vi "MC-21C Driver_simple.vi"(8 "Step":string="200", 9 "Operation":enum16{"forward", "backward", "stop"}(ring), 10 "Address":u8=1, 11 "Peristaltic Pump COM":refnum<visa-resource-name>="COM3") -> (2 "Write buffer":string)   [LabVIEW 2023]
panel:
  out "Read buffer":string
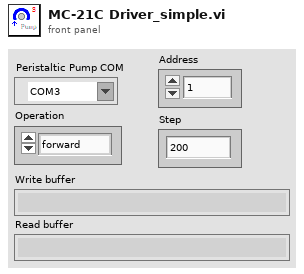
[diagram p1: front panel]
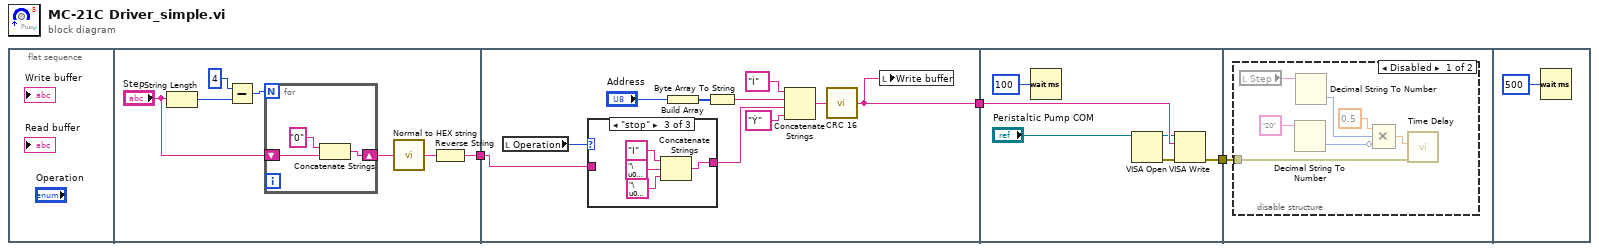
[diagram p0: block diagram]
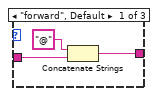
[diagram p2: hidden frame]
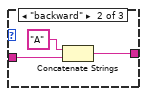
[diagram p3: hidden frame]
diagram:
  n1 = flat-sequence {
    tunnel: [w4] -> w3
    tunnel: w3 -> [w23]
    tunnel: [w14] -> w2
    tunnel: w2 -> [w37]
    tunnel: [w34] -> w1
    tunnel: w1 -> [w40]
    frame #0 {
    }
    frame #1 {
      n2 = String Length(string="Step") -> (length=w7:i32)
      n3 = Subtract(x=4, y=w7) -> (x-y=w8:i32)
      n4 = for {
        N: w8 -> [_]
        shift-right: [w11] -> w10
        shift-left: "Step" -> [w13]
        n5 = Concatenate Strings("0" ("string"), w13) -> (w11:string)
      }
      n6 = call "Normal to HEX string.vi"("input normal string"=w10) -> ("output HEX string"=w6:string)
      n7 = Reverse String(1:w6) -> (0:w4:string)
    }
    frame #2 {
      n8 = local read "Operation"() -> (w18:enum16{"forward", "backward", "stop"})
      n9 = case shown="\"stop\"" w18 {
        tunnel: w23 -> [w25 w28 _]
        tunnel: [w24 w27 w30] -> w17
        frame "forward", Default {
          n10 = Concatenate Strings("@" ("string"), w25) -> (w24:string)
        }
        frame "backward" {
          n11 = Concatenate Strings("A" ("string"), w28) -> (w27:string)
        }
        frame "stop" {
          n12 = Concatenate Strings("I" ("string"), "\u0000" ("string"), "\u0000" ("string")) -> (w30:string)
        }
      }
      n13 = Build Array("Address") -> (w21:u8[])
      n14 = Byte Array To String(unsigned byte array=w21) -> (string=w19:string)
      n15 = Concatenate Strings("Ì" ("string"), w19, w17, "Ý" ("string")) -> (w15:string)
      n16 = call "CRC 16.vi"("input HEX string"=w15) -> ("output HEX string"=w14:string)
      n17 = local write "Write buffer"(w14) -> ()
    }
    frame #3 {
      n18 = Wait (ms)(milliseconds to wait=u32 100) -> ()  [unwired: 1 out]
      n19 = VISA Open(VISA resource name="Peristaltic Pump COM") -> (VISA resource name=w35:refnum<visa-resource-name>, error out=w38:errorcluster)  [unwired: 4 in]
      n20 = VISA Write(VISA resource name=w35, write buffer=w37, error in (no error)=w38) -> (error out=w34:errorcluster)  [unwired: 2 out]
    }
    frame #4 {
      n21 = disable-structure shown="Disabled" {
        disable-tunnel: w40 -> [w47 _]
        frame Disabled {
          n22 = local read "Step"() -> (w45:string)
          n23 = Decimal String To Number(string="20") -> (number=w42:i32)  [unwired: 2 in, 1 out]
          n24 = Decimal String To Number(string=w45) -> (number=w43:i32)  [unwired: 2 in, 1 out]
          n25 = Compound Arithmetic op=MULTIPLY(0.5 ("value"), w43, invert w42) -> (w41:dbl)
          n26 = call "Time Delay"("error in (no error)"=w47, "Delay Time (s)"=w41) -> ()  [unwired: 9 in, 1 out]
        }
        frame Enabled {
        }
      }
    }
    frame #5 {
      n27 = Wait (ms)(milliseconds to wait=u32 500) -> ()  [unwired: 1 out]
    }
  }
